vi "AlliGator Get Image Destination File Path.vi"(6 "Image File Extension":string, 7 "Image Name Prefix":string, 8 "Error In":errorcluster, 9 "Current Data Set":i32, 10 "Time-Series Paths":path[](array[path]), 11 "Single Data Point Path":path) -> (0 "Error Out":errorcluster, 3 "Image File Path":path)   [LabVIEW 2021, in "AlliGator Source Image.lvlib"]
doc: "Builds path to save a front panel object's image based on its source and the current dataset."
uses:
  AlliGator Source Image.lvlib
  Files/AlliGator Files.lvlib
panel:
  # "see the AlliGator License on the block diagram (Ctrl+E or Window:Show Block Diagram)"
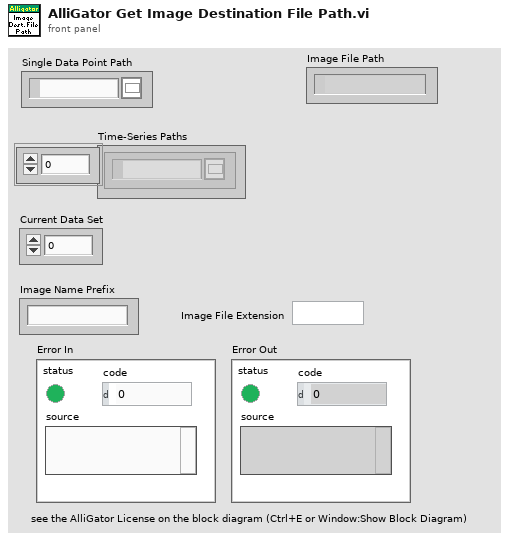
[diagram p1: front panel]
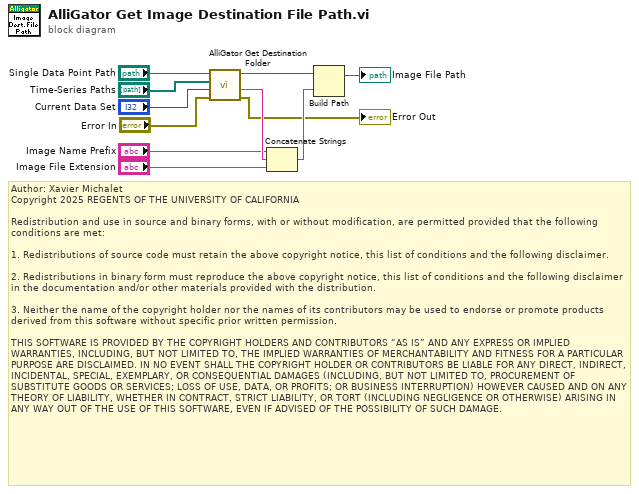
[diagram p0: block diagram]
diagram:
  # "Author: Xavier Michalet\nCopyright 2025 REGENTS OF THE UNIVERSITY OF CALIFORNIA\n\nRedistribution and use in source and binary forms, with or without modification, are permitted provided that the following conditions are met:\n\n1. Redistributions of source code must retain the above copyright notice, this list of conditions and the following disclaimer.\n\n2. Redistributions in binary form must reproduce the above copyright notice, this list of conditions and the following disclaimer in the documentation and/or other materials provided with the distribution.\n\n3. Neither the name of the copyright holder nor the names of its contributors may be used to endorse or promote products derived from this software without specific prior written permission.\n\nTHIS SOFTWARE IS PROVIDED BY THE COPYRIGHT HOLDERS AND CONTRIBUTORS “AS IS” AND ANY EXPRESS OR IMPLIED WARRANTIES, INCLUDING, BUT NOT LIMITED TO, THE IMPLIED WARRANTIES OF MERCHANTABILITY AND FITNESS FOR A PARTICULAR PURPOSE ARE DISCLAIMED. IN NO EVENT SHALL THE COPYRIGHT HOLDER OR CONTRIBUTORS BE LIABLE FOR ANY DIRECT, INDIRECT, INCIDENTAL, SPECIAL, EXEMPLARY, OR CONSEQUENTIAL DAMAGES (INCLUDING, BUT NOT LIMITED TO, PROCUREMENT OF SUBSTITUTE GOODS OR SERVICES; LOSS OF USE, DATA, OR PROFITS; OR BUSINESS INTERRUPTION) HOWEVER CAUSED AND ON ANY THEORY OF LIABILITY, WHETHER IN CONTRACT, STRICT LIABILITY, OR TORT (INCLUDING NEGLIGENCE OR OTHERWISE) ARISING IN ANY WAY OUT OF THE USE OF THIS SOFTWARE, EVEN IF ADVISED OF THE POSSIBILITY OF SUCH DAMAGE."
  n1 = call "AlliGator Get Destination Folder.vi"("Error In"="Error In", "Current Data Set (-1: single)"="Current Data Set", "Time-Series Paths"="Time-Series Paths", "Single Data Point Path"="Single Data Point Path") -> ("Error Out"=→"Error Out":errorcluster, "Data Point Name"=w11:string, "Destination Folder path"=w4:path)  [unwired: 5 in]
  n2 = Concatenate Strings("Image Name Prefix", w11, "Image File Extension") -> (w5:string)
  n3 = Build Path(base path=w4, name or relative path=w5) -> (appended path=→"Image File Path":path)
